vi "Update subpanel base path.vi"(8 "error in (no error)":errorcluster) -> (0 "error out":errorcluster)   [LabVIEW 2020]
uses:
  <userlib>/_MGI/Application Control/MGI Change Detector/MGI Change Detector (T).vi
  Global Variables/gl_Subpanel VI ref.vi
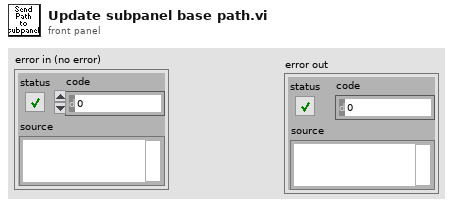
[diagram p1: front panel]
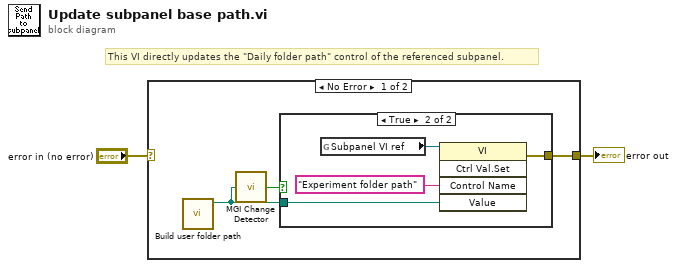
[diagram p0: block diagram]
diagram:
  # "This VI directly updates the \"Daily folder path\" control of the referenced subpanel."
  n1 = case shown="No Error" "error in (no error)" {
    selector: "error in (no error)" -> [_ w10]
    tunnel: [w4 w10] -> w2
    frame No Error {
      n2 = call "Build user folder path.vi"() -> ("Daily folder path with user folder appended?"=w3:path)  [unwired: 11 in]
      n3 = call-poly <userlib>:"MGI Change Detector.vi"("Value"=w3) -> ("Changed?"=w5:bool)
      n4 = case shown="True" w5 {
        tunnel: w3 -> [_ w9]
        tunnel: [_ w8] -> w4
        frame False {
        }
        frame True {
          n5 = global read "gl_Subpanel VI ref.vi" "Subpanel VI ref"() -> (w7:refnum<vi>)
          n6 = invoke class="VI" method="Ctrl Val.Set"(reference=w7, "Control Name"="Experiment folder path", "Value"=w9) -> (error out=w8:errorcluster)  [unwired: 2 in, 4 out]
        }
      }
    }
    frame Error {
    }
  }
  "error out" <- w2
